vi "Enviar_comando.vi"(8 "error in (no error)":errorcluster, 10 "Enum":T1, 11 "VISA resource name":refnum<visa-resource-name>) -> (0 "error out":errorcluster, 1 "return count":u32, 3 "VISA resource name out":refnum<visa-resource-name>)   [LabVIEW 2019]
uses:
  Typedefs/Comandos.ctl
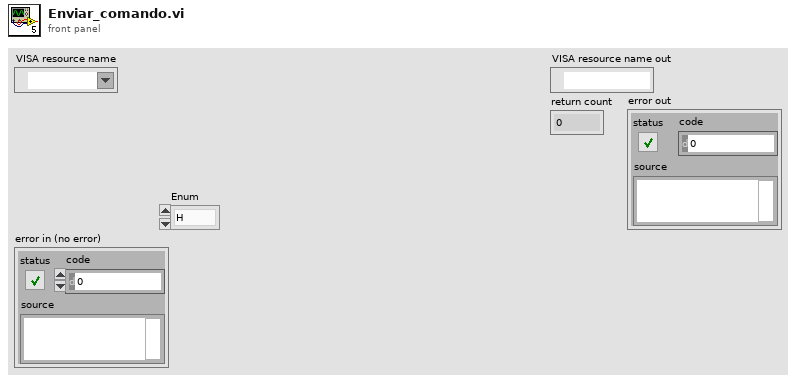
[diagram p1: front panel]
types:
  T1 = typedef "Comandos.ctl" = enum16{"H", "FH", "FM", "FI", "FX", "FY", "FZ", "I", "OK"}
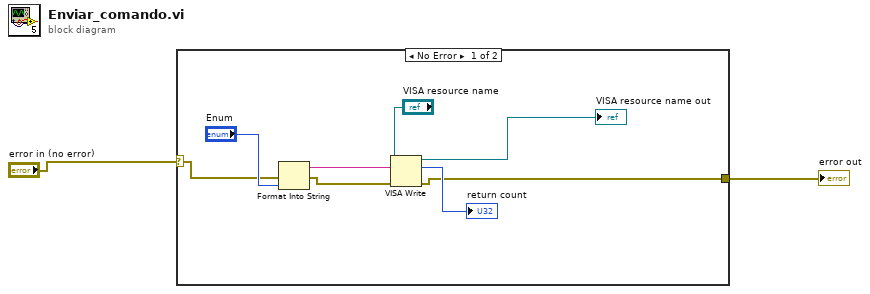
[diagram p0: block diagram]
diagram:
  n1 = case shown="No Error" "error in (no error)" {
    selector: "error in (no error)" -> [w5 w11]
    tunnel: [w3 w11] -> w1
    frame No Error {
      n2 = Format Into String(error in=w5, "Enum") -> (resulting string=w8:string, error out=w4:errorcluster)  [unwired: 2 in]
      n3 = VISA Write(VISA resource name="VISA resource name", write buffer=w8, error in (no error)=w4) -> (VISA resource name out=→"VISA resource name out":refnum<visa-resource-name>, return count=→"return count":u32, error out=w3:errorcluster)
    }
    frame Error {
    }
  }
  "error out" <- w1
